vi "Get Command Specifier.vi"(8 "error in":errorcluster, 11 "CANopen Message in":refnum<class "CANopen Message.lvclass">) -> (0 "error out":errorcluster, 2 "Command Specifier":u8 format="%.0x", 3 "CANopen Message out":refnum<class "CANopen Message.lvclass">)   [LabVIEW 2020, in "CANopen.lvlib" / "CANopen Message.lvclass"]
uses:
  CANopen Message.lvclass
  CANopen Message.lvclass/CANopen Message.ctl
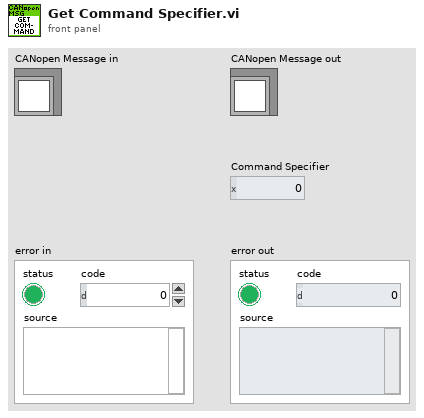
[diagram p1: front panel]
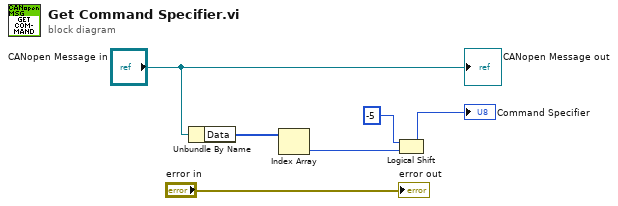
[diagram p0: block diagram]
diagram:
  n1 = Unbundle By Name("CANopen Message in") -> ("Data"=w5:u8[])
  n2 = Index Array(array=w5) -> (element=w3:u8)  [unwired: 1 in]
  n3 = Logical Shift(y=i16 -5, x=w3) -> (x << y=→"Command Specifier":u8)
  "CANopen Message out" <- "CANopen Message in"
  "error out" <- "error in"
